vi "Elevator Control Loop.vi"(11 "notifier":refnum<notifier>) -> ()   [LabVIEW 2019]
uses:
  Typedef/Controller Message.ctl
  <vilib>/Rock Robotics/WPI/MotorControl/WPI_MotorControlDeviceRef.ctl
  <vilib>/Rock Robotics/WPI/MotorControl/WPI_MotorControlType.ctl
  <vilib>/Rock Robotics/SystemInterfaces/DIO/FPGA_DIOPWMChannel.ctl
  <vilib>/Rock Robotics/WPI/PWM/WPI_PWMDeadband.ctl
  <vilib>/Rock Robotics/SystemInterfaces/DIO/FPGA_DIOChannel.ctl
  <vilib>/Rock Robotics/WPI/Encoder/WPI_EncoderDevRef.ctl
  <vilib>/Rock Robotics/SystemInterfaces/Encoder/FPGA_EncoderIdx.ctl
  <vilib>/Rock Robotics/SystemInterfaces/Counter/FPGA_CounterCtrSystemIndex.ctl
  <vilib>/Rock Robotics/WPI/Encoder/WPI_EncoderType.ctl
  <vilib>/Rock Robotics/WPI/DigitalInput/WPI_DigitalInputDevRef.ctl
  <vilib>/Platform/TimedLoop/XDataNode/timing_clust.ctl
  <vilib>/Platform/TimedLoop/XDataNode/nitl_modes.ctl
  <vilib>/Platform/TimedLoop/XDataNode/wakeup.ctl
  Typedef/FGVAction.ctl
  <vilib>/platform/TimedLoop/XDataNode/XDataNode.xnode
  <vilib>/Platform/TimedLoop/XDataNode/XDNodeRunTimeDep.lvlib
panel:
  in  "Position Max":dbl=100.0 format="%#_13g"
  in  "homing speed":dbl=0.05 format="%#_13g"
  in  "min speed":dbl=0.05 format="%#_13g"
  in  "gravity":dbl=0.15 format="%#_13g"
  in  "PIDF gains":cluster{"Kp":dbl, "Ki":dbl, "Kd":dbl, "Kf":dbl}={"Kp"=0.01, "Ki"=0.0, "Kd"=0.06, "Kf"=0.0} {"Kf" format="%.5f"; "Kd" format="%.3f"; "Ki" format="%.3f"; "Kp" format="%.3f"}
  out "Plant Input":T1(graph)
  in  "output range":cluster{"output high":dbl, "output low":dbl}={"output high"=1.0, "output low"=-1.0} {"output low" format="%.2f"; "output high" format="%.2f"}
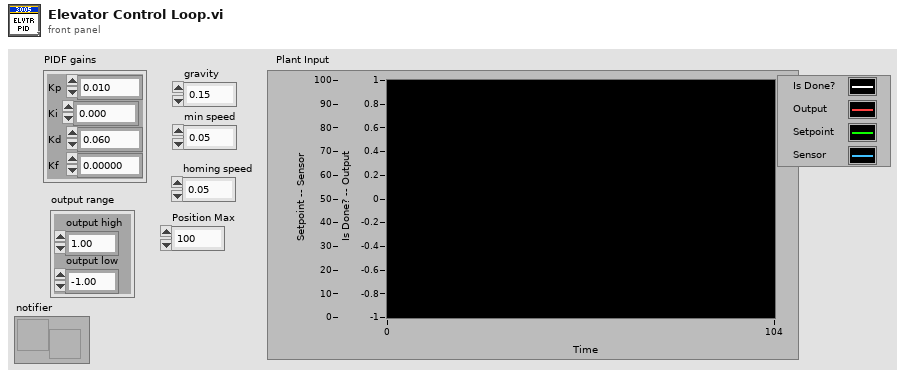
[diagram p1: front panel]
types:
  T1 = cluster{i16, dbl, "Setpoint":dbl, "Distance":dbl}
  T2 = typedef "WPI_MotorControlDeviceRef.ctl" = cluster{"DeviceStatus":errorcluster, "Type":T3, "PWM":cluster{"PWM Channel":T4, "DeadBand":T5}, "CAN":cluster{"Device Number":u8, "SetOutput VI Ref":variant, "GetOutput VI Ref":variant, "Enable VI Ref":variant, "Disable VI Ref":variant, "Data":variant}, "Invert":bool, "DIO PWM":cluster{"PWM \"Enable\" Channel":T4, "DIOChannel":T6, "PWM Rate":dbl}}
  T3 = typedef "WPI_MotorControlType.ctl" = enum16{"PWM", "CAN", "DIO PWM"}
  T4 = typedef "FPGA_DIOPWMChannel.ctl" = enum8{"PWM 0", "PWM 1", "PWM 2", "PWM 3", "PWM 4", "PWM 5", "PWM 6", "PWM 7", "PWM 8", "PWM 9", "PWM MXP 0", "PWM MXP 1", "PWM MXP 2", "PWM MXP 3", "PWM MXP 4", "PWM MXP 5", "PWM MXP 6", "PWM MXP 7", "PWM MXP 8", "PWM MXP 9", "Invalid"}
  T5 = typedef "WPI_PWMDeadband.ctl" = cluster{"Name":string, "maxPositivePwm":i32, "minPositivePwm":i32, "centerPwm":i32, "maxNegativePwm":i32, "minNegativePwm":i32, "angularRange":u16}
  T6 = typedef "FPGA_DIOChannel.ctl" = enum8{"DIO 0", "DIO 1", "DIO 2", "DIO 3", "DIO 4", "DIO 5", "DIO 6", "DIO 7", "DIO 8", "DIO 9", "DIO MXP 0", "DIO MXP 1", "DIO MXP 2", "DIO MXP 3", "DIO MXP 4", "DIO MXP 5", "DIO MXP 6", "DIO MXP 7", "DIO MXP 8", "DIO MXP 9", "DIO MXP 10", "DIO MXP 11", "DIO MXP 12", "DIO MXP 13", "DIO MXP 14", "DIO MXP 15", "SPI Port CS1", "SPI Port CS2", "SPI Port CS3", "SPI Port MISO", "SPI Port MOSI", "Invalid"}
  T7 = typedef "WPI_EncoderDevRef.ctl" = cluster{"DevStatus":errorcluster, "EncoderIndex":T8, "CounterIndex":T9, "DistancePerCount":dbl, "Decoding Type":T10}
  T8 = typedef "FPGA_EncoderIdx.ctl" = enum8{"Enc 0", "Enc 1", "Enc 2", "Enc 3", "Enc 4", "Enc 5", "Enc 6", "Enc 7", "Invalid"}
  T9 = typedef "FPGA_CounterCtrSystemIndex.ctl" = enum8{"Ctr 0", "Ctr 1", "Ctr 2", "Ctr 3", "Ctr 4", "Ctr 5", "Ctr 6", "Ctr 7", "Invalid"}
  T10 = typedef "WPI_EncoderType.ctl" = enum16{"1x", "2x", "4x"}
  T11 = typedef "WPI_DigitalInputDevRef.ctl" = cluster{"DevStatus":errorcluster, "DIO Channel":T6}
  T12 = cluster{"Setpoint":dbl, "Output":dbl, "DriveMotor1":T2, "Encoder":T7, "notifier":refnum<notifier>, "DriveMotor2":T2, "Top SW":T11, "Bottom SW":T11}
  T13 = typedef "XDNodeRunTimeDep.lvlib/timing_clust.ctl" = cluster{"Expected End [f-1]":u64, "Actual End [f-1]":u64, "Finished Late? [f-1]":bool, "Expected End [i-1]":u64, "Actual End [i-1]":u64, "Finished Late? [i-1]":bool, "Expected Start [i]":u64, "Actual Start [i]":u64, "Expected Start [f]":u64, "Actual Start [f]":u64, "Source Name":string, "Structure Name":string, "Period":i64, "Deadline":i64, "Offset":i64, "Start":i64, "Priority":i32, "Timeout":i32, "Mode":T14, "Wakeup Reason":T15, "Error":errorcluster, "Source Type":string, "Secondary Source Type":string, "Global End Time":u64, "Global Start Time":u64, "Frame Duration":u64, "Iteration Duration":u64, "Assigned CPU":i32, "I/O Scan Engine Mode":u32}
  T14 = typedef "XDNodeRunTimeDep.lvlib/nitl_modes.ctl" = enum32{"No Change", "Process missed periods, maintain original phase", "Discard missed periods, maintain original phase", "Process missed periods, ignore original phase", "Discard missed periods, ignore original phase"}
  T15 = typedef "XDNodeRunTimeDep.lvlib/wakeup.ctl" = enum32{"Normal", "Aborted", "Asynchronous wakeup", "Timing source error", "Timed loop error", "Timeout"}
  T16 = typedef "FGVAction.ctl" = enum16{"get", "set"}
  T17 = typedef "Controller Message.ctl" = cluster{"Setpoint":dbl, "Manual":bool}
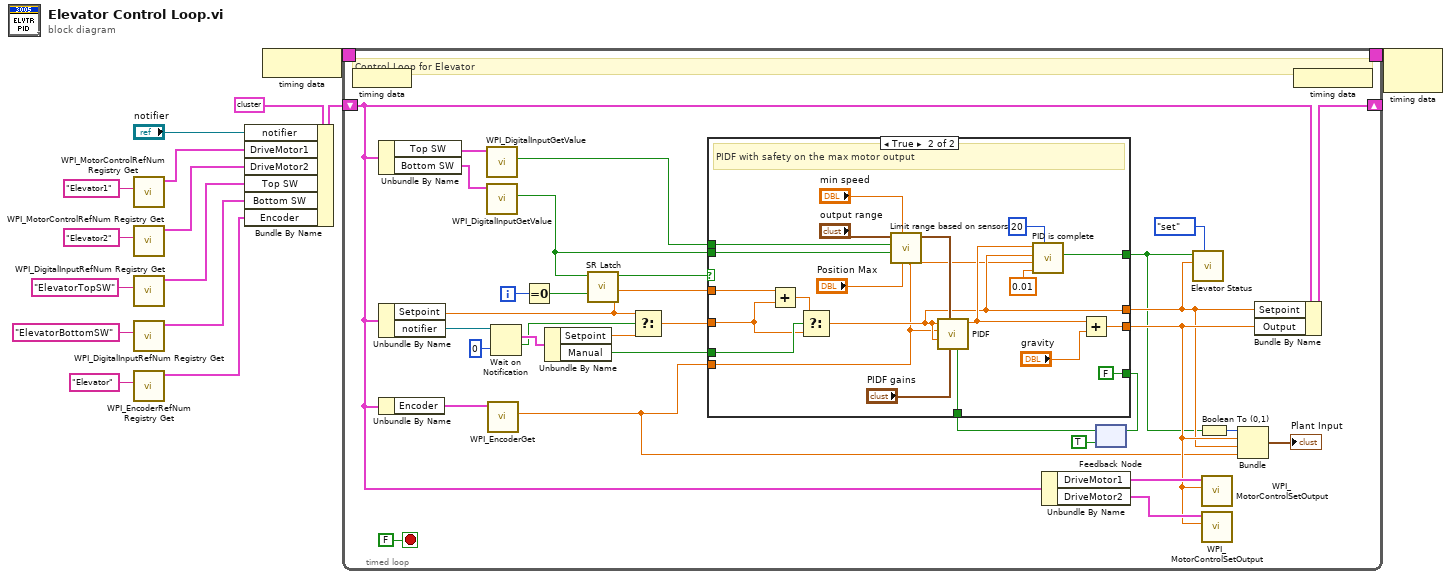
[diagram p0: block diagram]
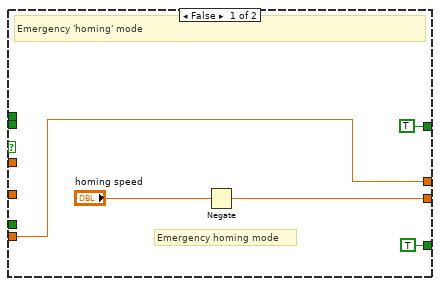
[diagram p2: hidden frame]
diagram:
  n1 = call <vilib>:"WPI_MotorControlRefNum Registry Get.vi"("refnum name"="Elevator1") -> ("MotorControlDevRef"=w6:T2)  [unwired: 9 in, 1 out]
  n2 = call <vilib>:"WPI_MotorControlRefNum Registry Get.vi"("refnum name"="Elevator2") -> ("MotorControlDevRef"=w5:T2)  [unwired: 9 in, 1 out]
  n3 = call <vilib>:"WPI_DigitalInputRefNum Registry Get.vi"("refnum name"="ElevatorTopSW") -> ("DigitalInputDevRef"=w4:T11)  [unwired: 9 in, 1 out]
  n4 = call <vilib>:"WPI_DigitalInputRefNum Registry Get.vi"("refnum name"="ElevatorBottomSW") -> ("DigitalInputDevRef"=w3:T11)  [unwired: 9 in, 1 out]
  n5 = call <vilib>:"WPI_EncoderRefNum Registry Get.vi"("refnum name"="Elevator") -> ("EncoderDevRef"=w2:T7)  [unwired: 9 in, 1 out]
  n6 = Bundle By Name(cluster=T12 {"Setpoint"=0.0, "Output"=0.0, "DriveMotor1"={"DeviceStatus"={"status"=FALSE, "code"=0, "source"=""}, "Type"=enum."PWM", "PWM"={"PWM Channel"=enum."Invalid", "DeadBand"={"Name"="", "maxPositivePwm"=0, "minPositivePwm"=0, "centerPwm"=0, "maxNegativePwm"=0, "minNegativePwm"=0, "angularRange"=0}}, "CAN"={"Device Number"=0, "SetOutput VI Ref"=variant(enum8{"Percent VBus", "Current", "Speed", "Position", "Voltage"} enum."Percent VBus"), "GetOutput VI Ref"=variant(refnum<k1> refnum), "Enable VI Ref"=variant(dbl 12.0), "Disable VI Ref"=variant(enum8{"Percent VBus", "Speed", "Position", "Slave", "Unchanged / Invalid"} enum."Percent VBus"), "Data"=variant(enum16{"Controller 1"} enum."Controller 1")}, "Invert"=FALSE, "DIO PWM"={"PWM \"Enable\" Channel"=enum."Invalid", "DIOChannel"=enum."Invalid", "PWM Rate"=0.0}}, "Encoder"={"DevStatus"={"status"=FALSE, "code"=0, "source"=""}, "EncoderIndex"=enum."Invalid", "CounterIndex"=enum."Invalid", "DistancePerCount"=1.0, "Decoding Type"=enum."4x"}, "notifier"=refnum, "DriveMotor2"={"DeviceStatus"={"status"=FALSE, "code"=0, "source"=""}, "Type"=enum."PWM", "PWM"={"PWM Channel"=enum."Invalid", "DeadBand"={"Name"="", "maxPositivePwm"=0, "minPositivePwm"=0, "centerPwm"=0, "maxNegativePwm"=0, "minNegativePwm"=0, "angularRange"=0}}, "CAN"={"Device Number"=0, "SetOutput VI Ref"=variant(enum8{"Percent VBus", "Current", "Speed", "Position", "Voltage"} enum."Percent VBus"), "GetOutput VI Ref"=variant(refnum<k1> refnum), "Enable VI Ref"=variant(dbl 12.0), "Disable VI Ref"=variant(enum8{"Percent VBus", "Speed", "Position", "Slave", "Unchanged / Invalid"} enum."Percent VBus"), "Data"=variant(enum16{"Controller 1"} enum."Controller 1")}, "Invert"=FALSE, "DIO PWM"={"PWM \"Enable\" Channel"=enum."Invalid", "DIOChannel"=enum."Invalid", "PWM Rate"=0.0}}, "Top SW"={"DevStatus"={"status"=FALSE, "code"=0, "source"=""}, "DIO Channel"=enum."Invalid"}, "Bottom SW"={"DevStatus"={"status"=FALSE, "code"=0, "source"=""}, "DIO Channel"=enum."Invalid"}}, "notifier"="notifier", "DriveMotor1"=w6, "DriveMotor2"=w5, "Top SW"=w4, "Bottom SW"=w3, "Encoder"=w2) -> (w14:T12)
  n7 = node-c288() -> (w13:T13)
  n8 = timed-loop {
    shift-right: [w44] -> _
    shift-left: w14 -> [w23]
    timing: w13 -> [_]
    timing-out: [_] -> w12
    i -> [w41]
    stop <- FALSE stop-if-true
    # "Control Loop for Elevator"
    n9 = node-c288() -> ()  [unwired: 1 in]
    n10 = Unbundle By Name(w23) -> ("Top SW"=w27:T11, "Bottom SW"=w26:T11)
    n11 = Unbundle By Name(w23) -> ("Setpoint"=w31:dbl, "notifier"=w45:refnum<notifier>)
    n12 = Unbundle By Name(w23) -> ("Encoder"=w22:T7)
    n13 = call <vilib>:"WPI_DigitalInputGetValue.vi"("DigitalInputDevRef"=w27) -> ("Value"=w25:bool)  [unwired: 8 in, 2 out]
    n14 = call <vilib>:"WPI_DigitalInputGetValue.vi"("DigitalInputDevRef"=w26) -> ("Value"=w24:bool)  [unwired: 8 in, 2 out]
    n15 = call <vilib>:"WPI_EncoderGet.vi"("EncoderDevRef"=w22) -> ("Distance"=w18:dbl)  [unwired: 5 in, 5 out]
    n16 = Wait on Notification(notifier=w45, timeout in ms (-1)=0) -> (notification=w35:T17, timed out?=w33:bool)  [unwired: 2 in, 2 out]
    n17 = Equal To 0?(x=w41) -> (x = 0?=w40:bool)
    n18 = Unbundle By Name(w35) -> ("Setpoint"=w34:dbl, "Manual"=w30:bool)
    n19 = call "SR Latch.vi"("Reset"=w40, "Value"=w24) -> ("Latched"=w32:bool)  [unwired: 7 in]
    n20 = Select(t=w31, s=w33, f=w34) -> (s? t:f=w42:dbl)
    n21 = Unbundle By Name(w23) -> ("DriveMotor1"=w29:T2, "DriveMotor2"=w28:T2)
    n22 = feedback #1(TRUE ("Reinitialize")) -> (w37:bool)
    n23 = case shown="True" w32 {
      tunnel: w42 -> [_ w56]
      tunnel: [w49 w67] -> w21
      tunnel: w25 -> [_ w65]
      tunnel: w24 -> [_ w64]
      tunnel: [w47 w53] -> w20
      tunnel: [TRUE ("PID is Done?") w63] -> w16
      tunnel: [TRUE ("Reinitialize") FALSE ("Reinitialize?")] -> w38
      tunnel: w37 -> [_ w62]
      tunnel: w30 -> [_ w60]
      tunnel: w31 -> [_ w58]
      tunnel: w18 -> [w47 w52]
      frame False {
        # "Emergency homing mode"
        # "Emergency 'homing' mode"
        n24 = Negate(x="homing speed") -> (-x=w49:dbl)
      }
      frame True {
        # "PIDF with safety on the max motor output"
        n25 = Add(x=w58, y=w56) -> (x+y=w59:dbl)
        n26 = Select(t=w59, s=w60, f=w56) -> (s? t:f=w53:dbl)
        n27 = call "Limit range based on sensors.vi"("Position"=w52, "Position Max"="Position Max", "min speed"="min speed", "Bottom SW"=w64, "Top SW"=w65, "output range in"="output range") -> ("output range out"=w69:cluster{"output high":dbl, "output low":dbl})  [unwired: 5 in]
        n28 = call "PIDF.vi"("reinitialize? (F)"=w62, "PIDF gains"="PIDF gains", "output range"=w69, "Feedforward"=w53, "process variable"=w52, "setpoint"=w53) -> ("output"=w71:dbl)  [unwired: 3 in, 2 out]
        n29 = call "PID is complete.vi"("sample length"=20, "threshold"=0.01, "process variable"=w52, "setpoint"=w53, "PID Output"=w71) -> ("PID is Done?"=w63:bool)  [unwired: 5 in, 1 out]
        n30 = Add(x=w71, y="gravity") -> (x+y=w67:dbl)
      }
    }
    n31 = feedback-in #1(w38) -> ()
    n32 = call "Elevator Status.vi"("Action"=FGVAction."set", "SP in"=w20, "Moving? (F)"=w16) -> ()  [unwired: 6 in, 3 out]
    n33 = Boolean To (0,1)(Boolean=w16) -> (0, 1=w17:i16)
    n34 = call <vilib>:"WPI_MotorControlSetOutput.vi"("Output"=w21, "MotorControlDevRef"=w29) -> ()  [unwired: 7 in, 3 out]
    n35 = call <vilib>:"WPI_MotorControlSetOutput.vi"("Output"=w21, "MotorControlDevRef"=w28) -> ()  [unwired: 7 in, 3 out]
    n36 = Bundle(w17, w21, "Setpoint"=w20, "Distance"=w18) -> (→"Plant Input":T1)  [unwired: 1 in]
    n37 = Bundle By Name(cluster=w23, "Setpoint"=w20, "Output"=w21) -> (w44:T12)
    n38 = node-c288() -> ()  [unwired: 1 out]
  }
  n39 = node-c288(w12) -> ()  [unwired: 1 out]
